vi "Split as Parent Child pair.vi"(0 "Functions":refnum<class "functionbase.lvclass">[](array[class]), 5 "Parent Indent":i64=-1, 11 "error in (no error)":errorcluster) -> (4 "Parent Child Combo":T1[](array[typedef]), 15 "error out":errorcluster)   [LabVIEW 2016]
uses:
  functions/functionsbase/functionbase.lvclass
  Function Indent Combo.ctl
  functions/functionsbase/functionbase.lvclass/functionbase.ctl
  functions/functionsbase/properties/Read Line#.vi
  functions/functionsbase/properties/Read Indent#.vi
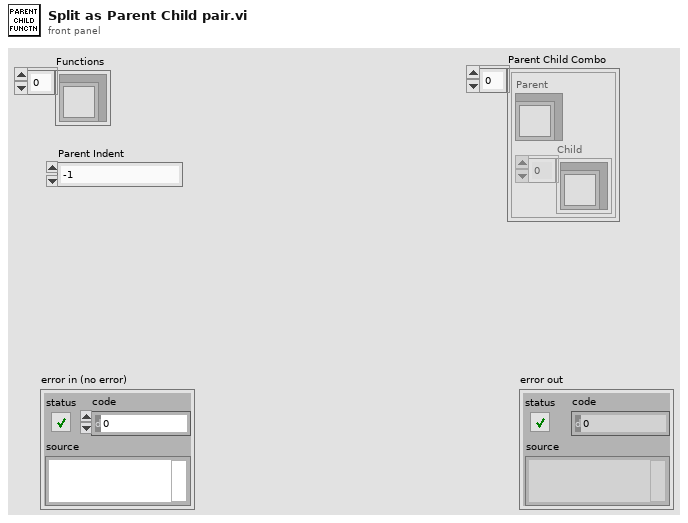
[diagram p1: front panel]
types:
  T1 = typedef "Function Indent Combo.ctl" = cluster{"Parent":refnum<class "functionbase.lvclass">, "Child":refnum<class "functionbase.lvclass">[]}
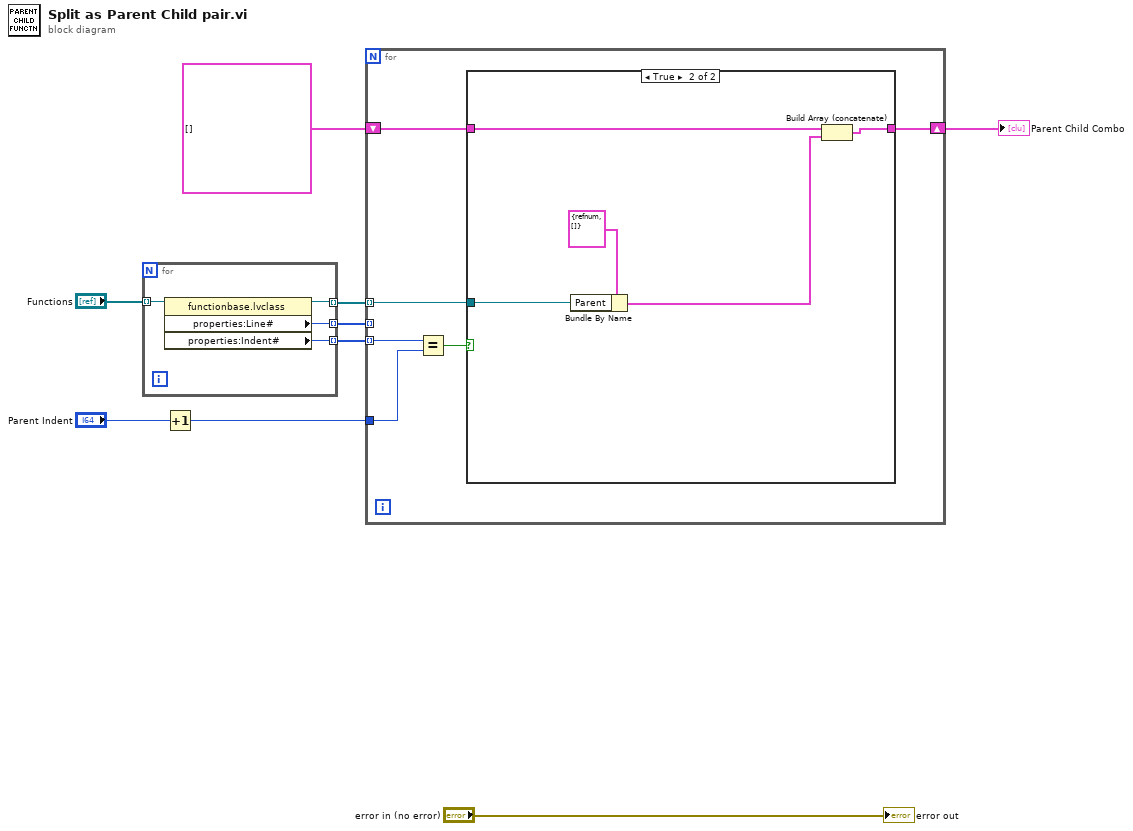
[diagram p0: block diagram]
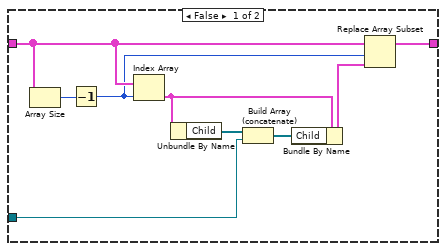
[diagram p2: hidden frame]
diagram:
  n1 = for {
    tunnel: "Functions" -> [w13] mode=indexing
    tunnel: [w12] -> w6 mode=indexing
    tunnel: [w11] -> w7 mode=indexing
    tunnel: [w10] -> w4 mode=indexing
    n2 = property class="functionbase.lvclass"(reference=w13) -> (reference out=w11:refnum<class "functionbase.lvclass">, "properties:Line#"=w12:i64, "properties:Indent#"=w10:i64)  [unwired: 1 in, 1 out]
  }
  n3 = Increment(x="Parent Indent") -> (x+1=w3:i64)
  n4 = for {
    shift-right: [w16] -> w2
    shift-left: T1[] [] -> [w18]
    tunnel: w7 -> [w17] mode=indexing
    tunnel: w6 -> [_] mode=indexing
    tunnel: w4 -> [w15] mode=indexing
    tunnel: w3 -> [w14]
    n5 = Equal?(x=w15, y=w14) -> (x = y?=w19:bool)
    n6 = case shown="True" w19 {
      tunnel: w18 -> [w26 w31]
      tunnel: w17 -> [w24 w32]
      tunnel: [w28 w29] -> w16
      frame False {
        n7 = Array Size(array=w26) -> (size(s)=w27:i32)
        n8 = Decrement(x=w27) -> (x-1=w20:i32)
        n9 = Index Array(array=w26, index=w20) -> (element=w23:T1)
        n10 = Unbundle By Name(w23) -> ("Child"=w25:refnum<class "functionbase.lvclass">[])
        n11 = Build Array (concatenate)(w25, w24) -> (w22:refnum<class "functionbase.lvclass">[])
        n12 = Bundle By Name(cluster=w23, "Child"=w22) -> (w21:T1)
        n13 = Replace Array Subset(array=w26, new element=w21, index=w20) -> (w28:T1[])
      }
      frame True {
        n14 = Bundle By Name(cluster=T1 {"Parent"=refnum, "Child"=[]}, "Parent"=w32) -> (w30:T1)
        n15 = Build Array (concatenate)(w31, w30) -> (w29:T1[])
      }
    }
  }
  "Parent Child Combo" <- w2
  "error out" <- "error in (no error)"
